vi "CRUD Create Example.vi"() -> ()   [LabVIEW 2020]
doc: "This performs an INSERT statement on the table that corresponds to bbPlayers. It will insert values for pName, pGames, pAverage, and pAvailable but will ignore the value provided for pNum. This assumes that pNum is the primary key and that it is an Identity, so that the database itself generates new values for it based on the values that already exist."
uses:
  BB Players Map/BB Players Map.lvclass
  BB Players/bbPlayers.lvclass
  f75d9549-9907-4d84-8846-08e249c265ff.vi
  <vilib>/Viviota/shared/ORM.lvlibp/ORM/SqlMapper/SqlMapper.lvclass
  <vilib>/Viviota/shared/ORM_DBC_Mssql.lvlibp/DBC.lvclass
panel:
  in  "pNum":i32
  in  "pAvailable":bool
  in  "pAverage":dbl
  in  "pGames":i32
  in  "pName":string
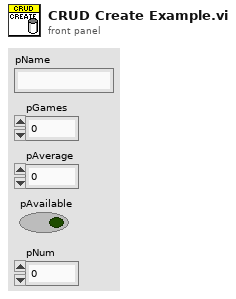
[diagram p1: front panel]
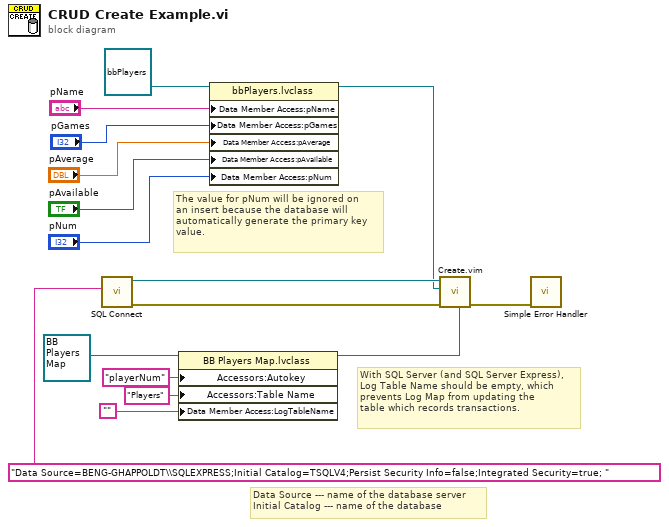
[diagram p0: block diagram]
diagram:
  # "The value for pNum will be ignored on\nan insert because the database will \nautomatically generate the primary key\nvalue."
  # "Data Source --- name of the database server\nInitial Catalog --- name of the database"
  # "With SQL Server (and SQL Server Express),\nLog Table Name should be empty, which\nprevents Log Map from updating the \ntable which records transactions."
  n1 = call <vilib>:"SQL Connect.vi"("Connection String"="Data Source=BENG-GHAPPOLDT\\SQLEXPRESS;Initial Catalog=TSQLV4;Persist Security Info=false;Integrated Security=true; ") -> ("error out"=w16:errorcluster, "SQL Mapper"=w14:refnum<class "SqlMapper.lvclass">)  [unwired: 9 in]
  n2 = property class="BB Players Map.lvclass"(reference=refnum<class "BB Players Map.lvclass"> refnum ("BB Players Map.lvclass"), "Accessors:Autokey"="playerNum" ("Autokey"), "Accessors:Table Name"="Players" ("Table Name"), "Data Member Access:LogTableName"="") -> (reference out=w6:refnum<class "BB Players Map.lvclass">)  [unwired: 1 in, 1 out]
  n3 = property class="bbPlayers.lvclass"(reference=refnum<class "bbPlayers.lvclass"> refnum ("bbPlayers.lvclass"), "Data Member Access:pName"="pName", "Data Member Access:pGames"="pGames", "Data Member Access:pAverage"="pAverage", "Data Member Access:pAvailable"="pAvailable", "Data Member Access:pNum"="pNum") -> (reference out=w10:refnum<class "bbPlayers.lvclass">)  [unwired: 1 in, 1 out]
  n4 = call "Create.vim"("TypeMap in"=w6, "error in (no error)"=w16, "object in"=w10, "SqlMapper in"=w14) -> ("error out"=w15:errorcluster)  [unwired: 4 in, 3 out]
  n5 = call <vilib>:"Simple Error Handler.vi"("error in (no error)"=w15) -> ()  [unwired: 4 in, 5 out]
